vi "MOD_STATE_FGV.vi"(7 "Write":bool, 8 "Right Dist":dbl, 9 "Right Speed":dbl, 10 "Left Dist":dbl, 11 "Left Speed":dbl) -> (0 "out Right Dist":dbl, 1 "out Right Speed":dbl, 2 "out Left Dist":dbl, 3 "out Left Speed":dbl)   [LabVIEW 2019]
panel:
  # "NON-REENTRANT\nON PURPOSE TO\nALLOW SAVING VALUES..."
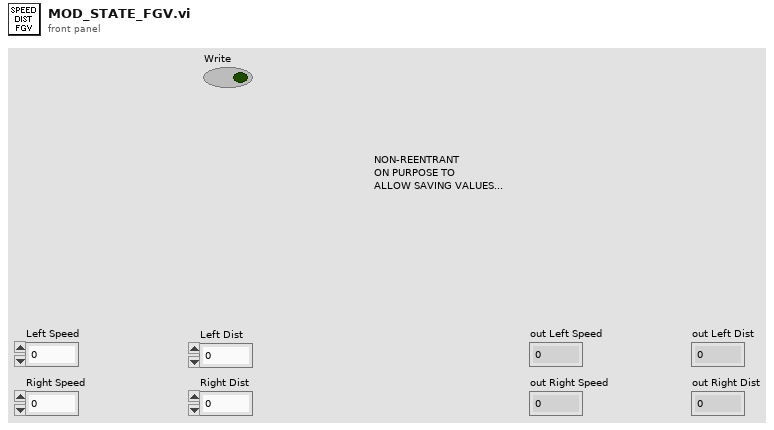
[diagram p1: front panel]
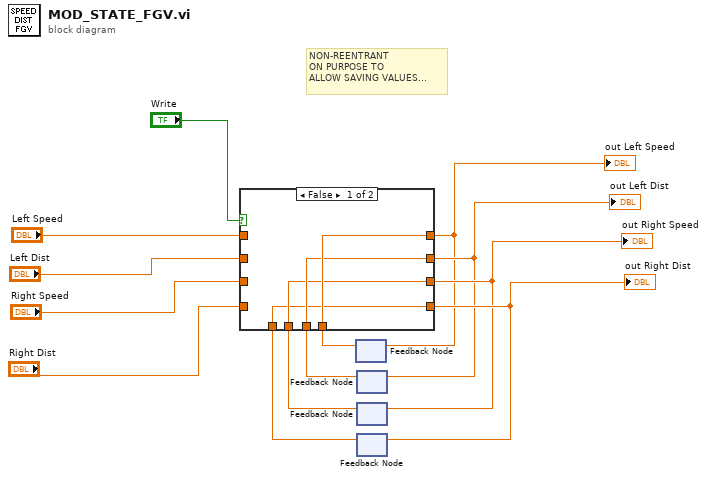
[diagram p0: block diagram]
diagram:
  # "NON-REENTRANT\nON PURPOSE TO\nALLOW SAVING VALUES..."
  n1 = feedback #1() -> (w10:dbl)  [unwired: 1 in]
  n2 = feedback #2() -> (w11:dbl)  [unwired: 1 in]
  n3 = feedback #3() -> (w12:dbl)  [unwired: 1 in]
  n4 = feedback #4() -> (w13:dbl)  [unwired: 1 in]
  n5 = case shown="False" "Write" {
    tunnel: "Left Speed" -> [_ w21]
    tunnel: "Left Dist" -> [_ w20]
    tunnel: "Right Speed" -> [_ w19]
    tunnel: "Right Dist" -> [_ w18]
    tunnel: [w17 w21] -> w6
    tunnel: [w16 w20] -> w7
    tunnel: [w15 w19] -> w8
    tunnel: [w14 w18] -> w9
    tunnel: w10 -> [w17 _]
    tunnel: w11 -> [w16 _]
    tunnel: w12 -> [w15 _]
    tunnel: w13 -> [w14 _]
    frame False {
    }
    frame True {
    }
  }
  "out Right Dist" <- w9
  "out Right Speed" <- w8
  "out Left Dist" <- w7
  "out Left Speed" <- w6
  n6 = feedback-in #1(w6) -> ()
  n7 = feedback-in #2(w7) -> ()
  n8 = feedback-in #3(w8) -> ()
  n9 = feedback-in #4(w9) -> ()
